vi "memoria.vi"() -> ()   [LabVIEW 2020]
uses:
  <vilib>/Analysis/2dsp.llb/1D Auto Correlation (DBL).vi
  <vilib>/Analysis/NI_AALPro.lvlib
panel:
  out "Rxx":dbl[][](array[numeric])
  out "normalizado":dbl[][](array[numeric])
  in  "Ruta":path
  out "firma":dbl[][](array[numeric])
  out "appended array":dbl[][](array[numeric])
  out "imagen":picture
  out "Firma de la imagen":dbl[](graph)
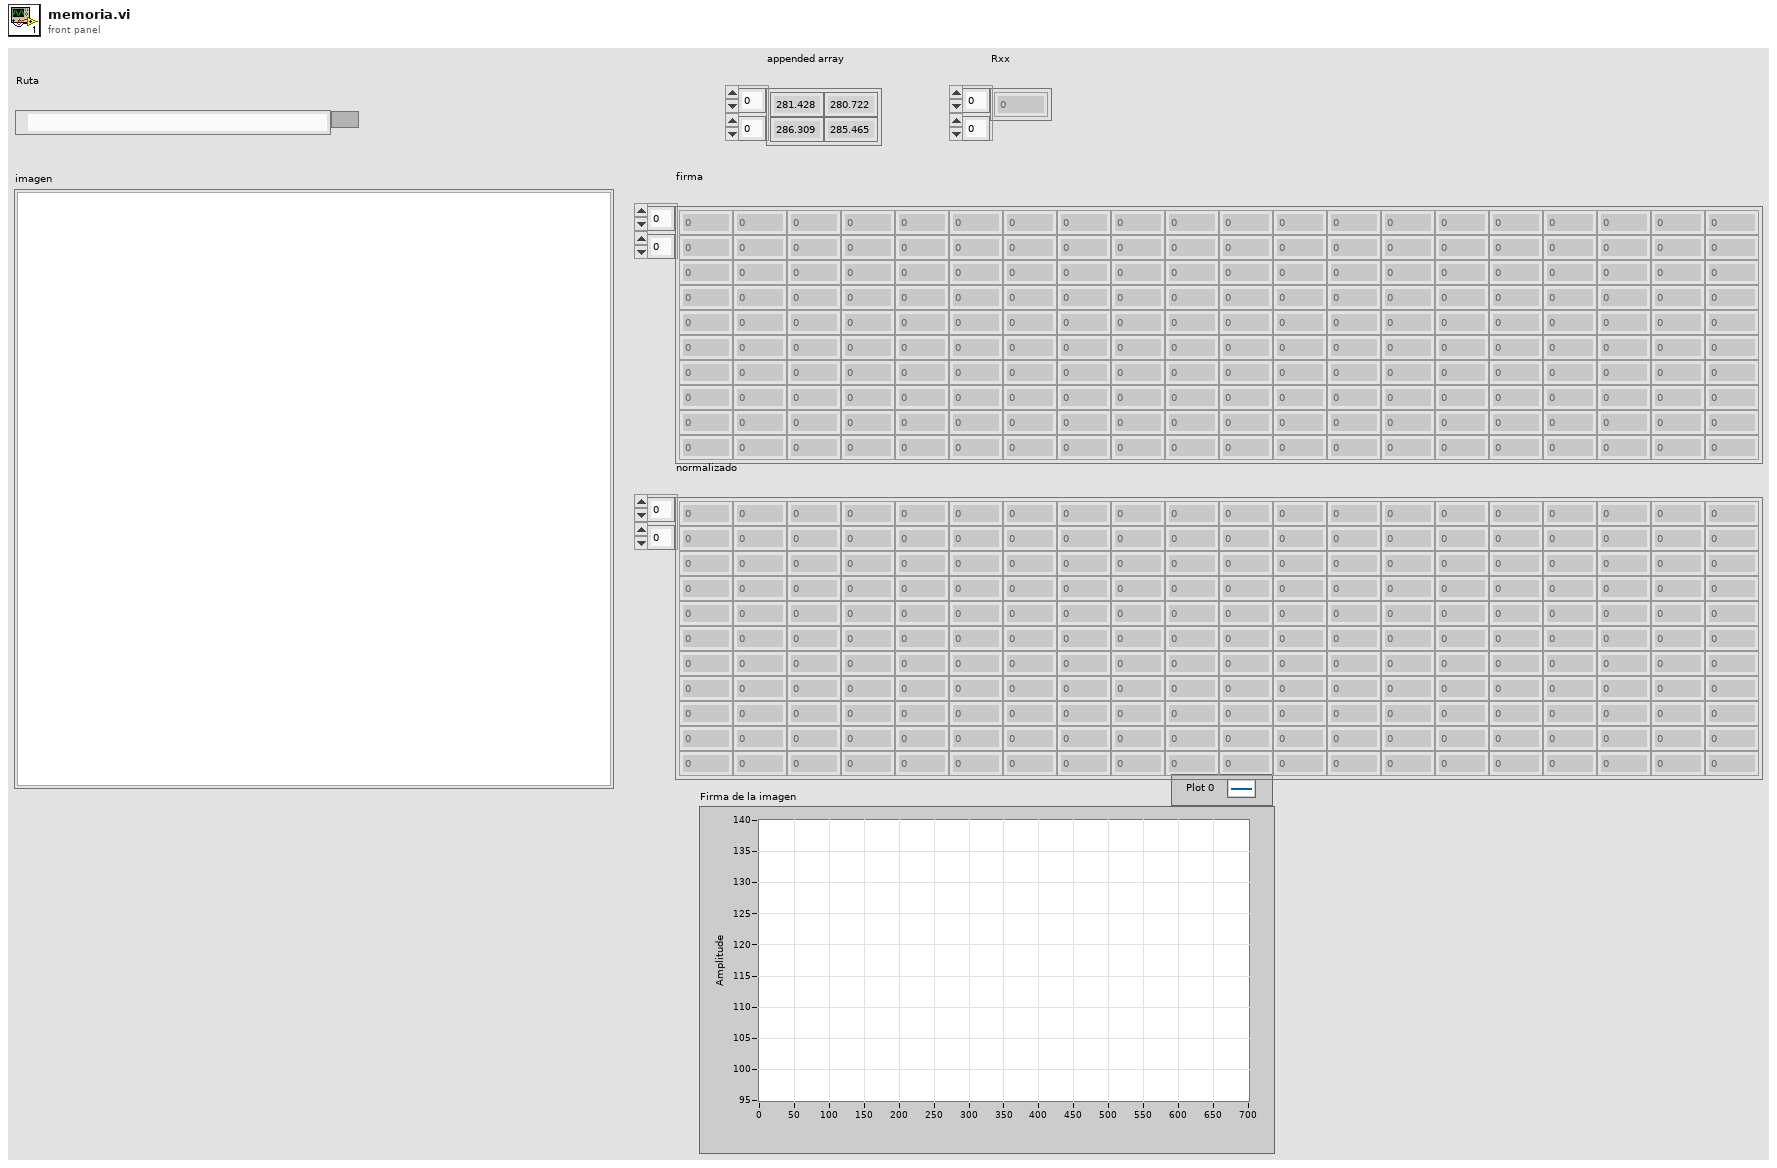
[diagram p1: front panel]
types:
  T1 = typedef "imagedata.ctl" = cluster{"image type":i32, "image depth":i32, "image":u8[], "mask":u8[], "colors":u32[], "Rectangle":cluster{"left":i16, "top":i16, "right":i16, "bottom":i16}}
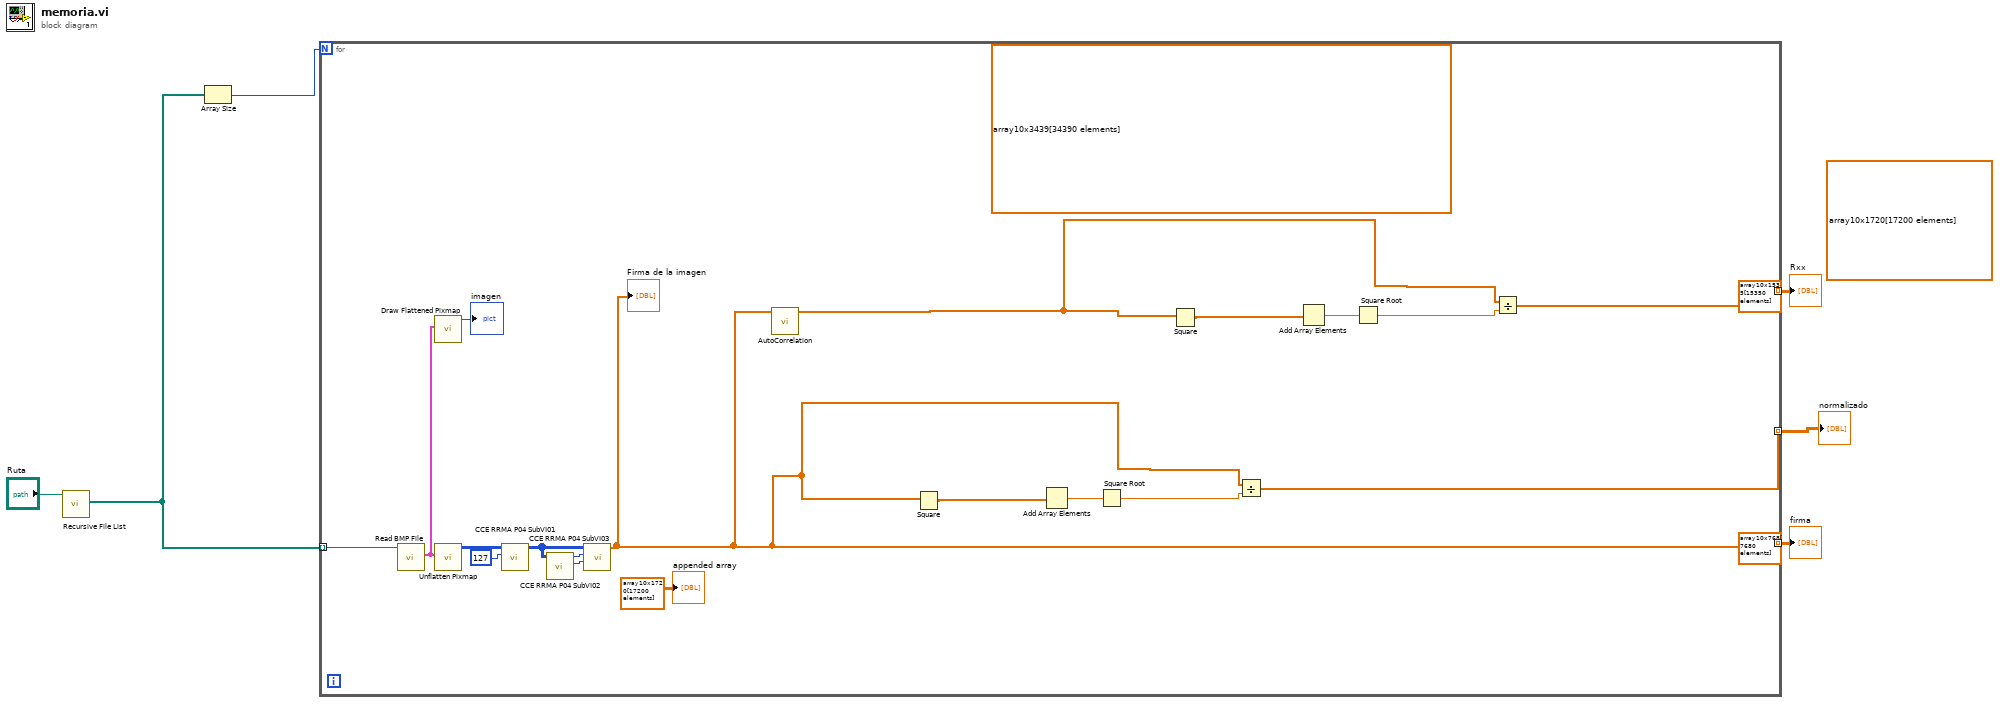
[diagram p0: block diagram]
diagram:
  (unwired) dbl[][] array10x768[7680 elements] ("firma")
  (unwired) dbl[][] array10x1535[15350 elements] ("Rxx")
  (unwired) dbl[][] array10x1720[17200 elements] ("normalizado")
  n1 = call <vilib>:"Recursive File List.vi"("Folder Path"="Ruta") -> ("All Files in Dir"=w3:path[])  [unwired: 6 in, 4 out]
  n2 = Array Size(array=w3) -> (size(s)=w4:i32)
  n3 = for {
    N: w4 -> [_]
    tunnel: w3 -> [w23] mode=indexing
    tunnel: [w12] -> w6 mode=indexing
    tunnel: [w13] -> w2 mode=indexing
    tunnel: [w8] -> w1 mode=indexing
    (unwired) dbl[][] array10x3439[34390 elements] ("Rxx")
    n4 = call <vilib>:"Read BMP File.vi"("path to BMP file"=w23) -> ("image data"=w24:T1)  [unwired: 8 in, 2 out]
    n5 = call <vilib>:"Draw Flattened Pixmap.vi"("image data"=w24) -> ("new picture"=→"imagen":picture)  [unwired: 8 in]
    n6 = call <vilib>:"Unflatten Pixmap.vi"("image data"=w24) -> ("24-bit pixmap"=w21:u32[][])  [unwired: 4 in, 6 out]
    n7 = call "CCE RRMA P04 SubVI01.vi"("24-bit pixmap"=w21, "umbral superior"=u32 127 ("umbral")) -> ("Array"=w20:u32[][])  [unwired: 8 in]
    n8 = call "CCE RRMA P04 SubVI02.vi"("Array"=w20) -> ("cy"=w18:u32, "cx"=w19:u32)  [unwired: 9 in]
    n9 = call "CCE RRMA P04 SubVI03.vi"("Cy"=w18, "Cx"=w19, "imagen"=w20) -> ("firma"=w12:dbl[])  [unwired: 8 in]
    "Firma de la imagen" <- w12
    n10 = call-poly <vilib>:"AutoCorrelation.vi"("X"=w12) -> ("Rxx"=w7:dbl[])  [unwired: 9 in, 1 out]
    n11 = Square(x=w12) -> (x^2=w15:dbl[])
    n12 = Add Array Elements(numeric array=w15) -> (sum=w16:dbl)
    n13 = Square Root(x=w16) -> (sqrt(x)=w14:dbl)
    n14 = Square(x=w7) -> (x^2=w10:dbl[])
    n15 = Divide(x=w12, y=w14) -> (x/y=w13:dbl[])
    n16 = Add Array Elements(numeric array=w10) -> (sum=w11:dbl)
    n17 = Square Root(x=w11) -> (sqrt(x)=w9:dbl)
    n18 = Divide(x=w7, y=w9) -> (x/y=w8:dbl[])
    "appended array" <- dbl[][] array10x1720[17200 elements] ("appended array")
  }
  "firma" <- w6
  "normalizado" <- w2
  "Rxx" <- w1
